vi "Get Result.vi"(8 "error in (no error)":errorcluster, 11 "ZI Lockin in":refnum<class "ZI Lockin.lvclass">) -> (0 "error out":errorcluster, 2 "Result":refnum<class "Acquired Result.lvclass">, 3 "ZI Lockin out":refnum<class "ZI Lockin.lvclass">)   [LabVIEW 2016, in "ZI Lockin.lvclass"]
uses:
  ZI Lockin.lvclass
  NHMFL_Core/Libraries/Instruments/Results/Acquired Result/Acquired Result.lvclass
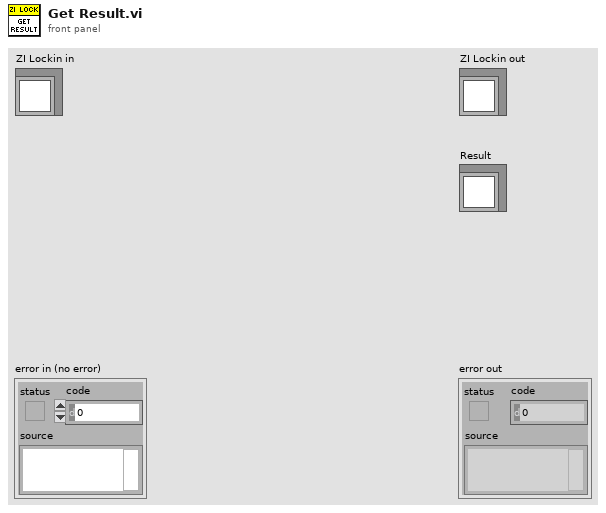
[diagram p1: front panel]
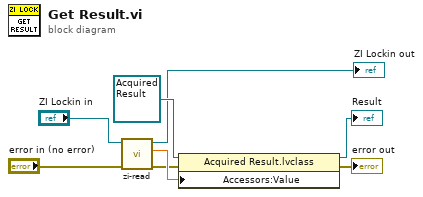
[diagram p0: block diagram]
diagram:
  n1 = call-dynamic "zi-read.vi"("error in (no error)"="error in (no error)", "ZI Lockin in"="ZI Lockin in") -> ("error out"=w1:errorcluster, "Result"=w2:dbl, "ZI Lockin out"=→"ZI Lockin out":refnum<class "ZI Lockin.lvclass">)  [unwired: 7 in]
  n2 = property class="Acquired Result.lvclass"(reference=refnum<class "Acquired Result.lvclass"> refnum ("Result"), error in=w1, "Accessors:Value"=w2) -> (reference out=→"Result":refnum<class "Acquired Result.lvclass">, error out=→"error out":errorcluster)
